vi "LVProjectShortcut_CreateShortcut.vi"(6 "error in":errorcluster, 9 "Wizard":T1) -> (0 "error out":errorcluster, 3 "Cancelled?":bool)   [LabVIEW 2017]
doc: "Use this template to create a wizard dialog."
uses:
  <resource>/Framework/Providers/API/ItemRef.ctl
  <resource>/Framework/Providers/API/mxLvChangeType.ctl
  <resource>/Framework/Providers/API/mxLvUpdateUI.ctl
panel:
  in  "Cancel":bool
  in  "OK Button":bool
  in  "Next":bool
  in  "Name":string caption="Type a name for this shortcut:"
  in  "File Path":path caption="Type the location of the item:"
  out "indication":string
  # "What item would you like to create a shortcut for?"
  # "This wizard helps you to create shortcut to files or folders."
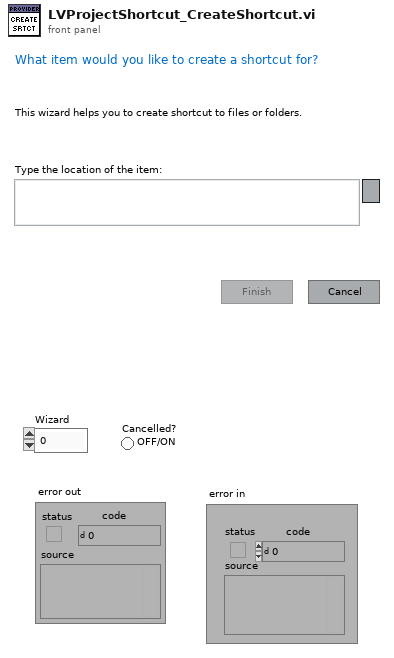
[diagram p1: front panel]
types:
  T1 = typedef "ItemRef.ctl" = u64
  T2 = enum8{"Enabled", "Disabled", "Disabled and Grayed Out"}
  T3 = typedef "mxLvUpdateUI.ctl" = cluster{"Action":u32, "Optional param 1":string, "Optional param 2":i32, "Optional param 3":string}
  T4 = typedef "mxLvChangeType.ctl" = enum32{"Item Created", "Item Modified", "File Modified", "File Deleted", "Item Added", "Item Added to SCC", "Item Renamed", "Item Modified For SCC"}
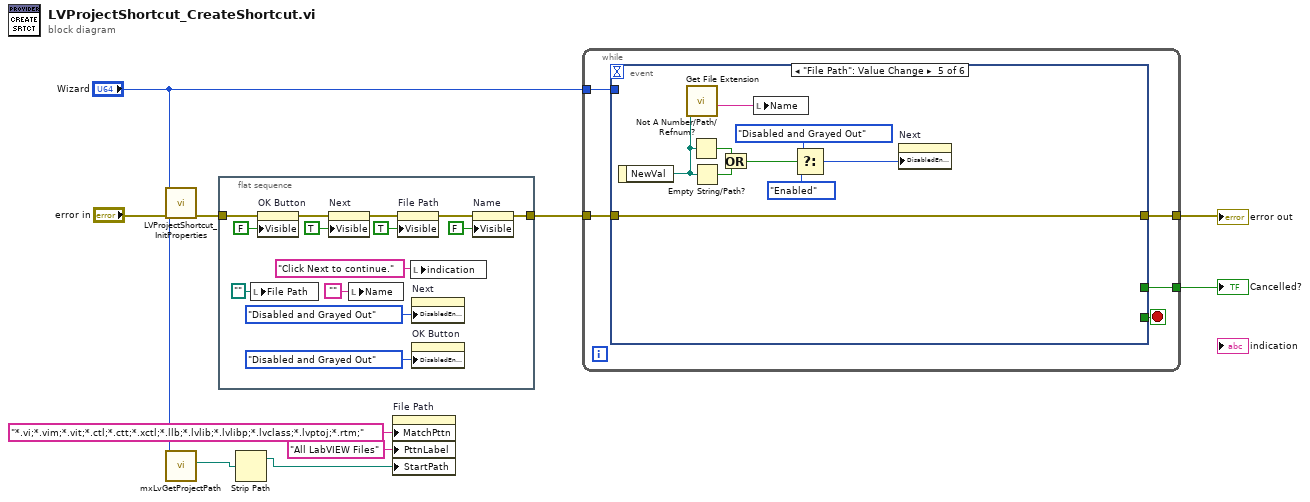
[diagram p0: block diagram]
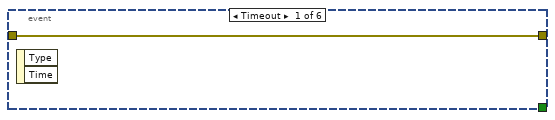
[diagram p2: hidden frame]
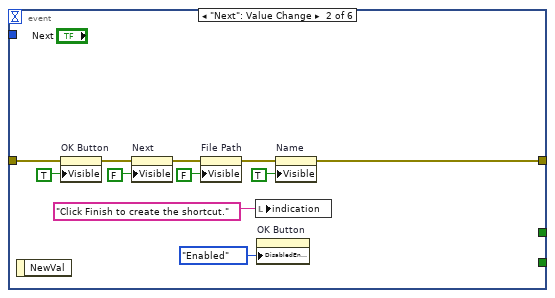
[diagram p3: hidden frame]
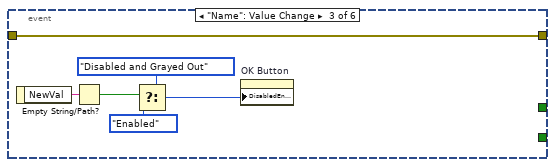
[diagram p4: hidden frame]
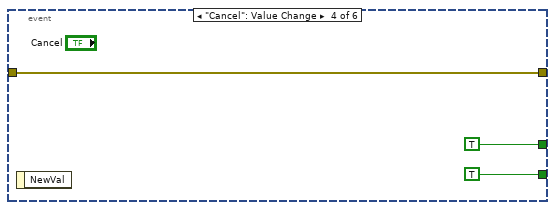
[diagram p5: hidden frame]
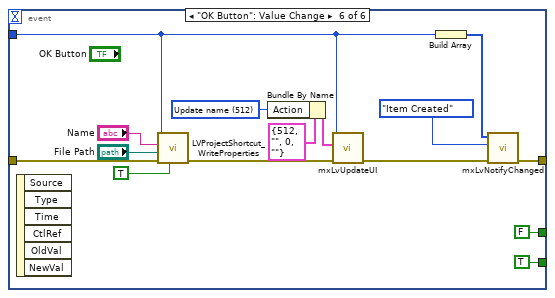
[diagram p6: hidden frame]
diagram:
  n1 = call <resource>:"LVProjectShortcut_InitProperties.vi"("error in"="error in", "Wizard"="Wizard") -> ("error out"=w6:errorcluster)  [unwired: 9 in]
  n2 = call <resource>:"mxLvGetProjectPath.vi"("Item"="Wizard") -> ("Project Path"=w2:path)  [unwired: 8 in, 2 out]
  n3 = flat-sequence {
    tunnel: w6 -> [w16]
    tunnel: [w15] -> w9
    frame #0 {
      n4 = local write "File Path"(path "") -> ()
      n5 = property on="OK Button" class="Bool"(error in=w16, "Visible"=FALSE) -> (error out=w19:errorcluster)  [unwired: 1 in, 1 out]
      n6 = property on="Next" class="Bool"(error in=w19, "Visible"=TRUE) -> (error out=w18:errorcluster)  [unwired: 1 in, 1 out]
      n7 = local write "Name"("") -> ()
      n8 = property on="File Path" class="Path"(error in=w18, "Visible"=TRUE) -> (error out=w17:errorcluster)  [unwired: 1 in, 1 out]
      n9 = local write "indication"("Click Next to continue.") -> ()
      n10 = property on="Next" class="Bool"("DisabledEnum"=T2."Disabled and Grayed Out" ("Disabled")) -> ()  [unwired: 2 in, 2 out]
      n11 = property on="OK Button" class="Bool"("DisabledEnum"=T2."Disabled and Grayed Out" ("Disabled")) -> ()  [unwired: 2 in, 2 out]
      n12 = property on="Name" class="Str"(error in=w17, "Visible"=FALSE) -> (error out=w15:errorcluster)  [unwired: 1 in, 1 out]
    }
  }
  n13 = Strip Path(path=w2) -> (stripped path=w1:path)  [unwired: 1 out]
  n14 = property on="File Path" class="Path"("MatchPttn"="*.vi;*.vim;*.vit;*.ctl;*.ctt;*.xctl;*.llb;*.lvlib;*.lvlibp;*.lvclass;*.lvptoj;*.rtm;" ("Browse Options:Match Pattern"), "PttnLabel"="All LabVIEW Files" ("Browse Options:Pattern Label"), "StartPath"=w1) -> ()  [unwired: 2 in, 2 out]
  n15 = while {
    tunnel: [w28] -> w10
    tunnel: w9 -> [w27]
    tunnel: [w26] -> w8
    tunnel: "Wizard" -> [w25]
    stop <- w29 stop-if-true
    n16 = event shown="[4] \"File Path\": Value Change" {
      selector: _ -> [_ _ _ _ _ _]
      dyn-events: _ -> [_ _ _ _ _ _]
      timeout: _ -> [_ _ _ _ _ _]
      tunnel: [_ _ _ TRUE _ TRUE] -> w29
      tunnel: [_ _ _ TRUE ("Cancelled?") _ FALSE ("Cancelled?")] -> w28
      tunnel: w27 -> [w30 w34 w42 w48 w53 w74]
      tunnel: [w30 w33 w42 w48 w53 w69] -> w26
      tunnel: w25 -> [_ _ _ _ _ w60]
      event Timeout {
        n17 = event-data() -> ()  [unwired: 1 in, 2 out]
      }
      event "Next": Value Change {
        n18 = event-data() -> ()  [unwired: 1 in, 1 out]
        n19 = property on="OK Button" class="Bool"(error in=w34, "Visible"=TRUE) -> (error out=w39:errorcluster)  [unwired: 1 in, 1 out]
        n20 = property on="Next" class="Bool"(error in=w39, "Visible"=FALSE) -> (error out=w40:errorcluster)  [unwired: 1 in, 1 out]
        n21 = property on="File Path" class="Path"(error in=w40, "Visible"=FALSE) -> (error out=w41:errorcluster)  [unwired: 1 in, 1 out]
        n22 = local write "indication"("Click Finish to create the shortcut.") -> ()
        n23 = property on="OK Button" class="Bool"("DisabledEnum"=T2."Enabled" ("Disabled")) -> ()  [unwired: 2 in, 2 out]
        n24 = property on="Name" class="Str"(error in=w41, "Visible"=TRUE) -> (error out=w33:errorcluster)  [unwired: 1 in, 1 out]
      }
      event "Name": Value Change {
        n25 = event-data() -> ("NewVal"=w47:string)  [unwired: 1 in]
        n26 = Empty String/Path?(string/path=w47) -> (empty?=w43:bool)
        n27 = Select(t=T2."Disabled and Grayed Out" ("Disabled"), s=w43, f=T2."Enabled" ("Disabled")) -> (s? t:f=w46:T2)
        n28 = property on="OK Button" class="Bool"("DisabledEnum"=w46) -> ()  [unwired: 2 in, 2 out]
      }
      event "Cancel": Value Change {
        n29 = event-data() -> ()  [unwired: 1 in, 1 out]
      }
      event "File Path": Value Change {
        n30 = event-data() -> ("NewVal"=w52:path)  [unwired: 1 in]
        n31 = call <vilib>:"Get File Extension.vi"("file"=w52) -> ("filename without extension"=w51:string)  [unwired: 6 in, 4 out]
        n32 = Not A Number/Path/Refnum?(number/path/refnum=w52) -> (NaN/Path/Refnum?=w59:bool)
        n33 = Empty String/Path?(string/path=w52) -> (empty?=w58:bool)
        n34 = Or(x=w59, y=w58) -> (x .or. y?=w57:bool)
        n35 = local write "Name"(w51) -> ()
        n36 = Select(t=T2."Disabled and Grayed Out" ("Disabled"), s=w57, f=T2."Enabled" ("Disabled")) -> (s? t:f=w54:T2)
        n37 = property on="Next" class="Bool"("DisabledEnum"=w54) -> ()  [unwired: 2 in, 2 out]
      }
      event "OK Button": Value Change {
        w65 = u32 512 items=["Do nothing"=0, "Browse to item"=1, "Update item state"=2, "Update item icon"=4, "Activate view"=8, "Update view list"=16, "Expand item"=32, "Update child list"=64, "Update help"=128, "Refresh item 'F5'"=256, "Update name"=512, "Update menus and toolbars"=1024, "Update all user interface"=1494] ("Action")
        n38 = event-data() -> ()  [unwired: 1 in, 6 out]
        n39 = call <resource>:"LVProjectShortcut_WriteProperties.vi"("hasPath"=TRUE, "error in"=w74, "filePath"="File Path", "shortcutName"="Name", "Wizard"=w60) -> ("error out"=w64:errorcluster)  [unwired: 6 in]
        n40 = Bundle By Name(cluster=T3 {"Action"=512, "Optional param 1"="", "Optional param 2"=0, "Optional param 3"=""} ("Update UI Settings"), "Action"=w65) -> (w61:T3)
        n41 = call <resource>:"mxLvUpdateUI.vi"("error in"=w64, "Update UI Settings"=w61, "Item"=w60) -> ("error out"=w63:errorcluster)  [unwired: 7 in, 1 out]
        n42 = Build Array(w60) -> (w68:T1[])
        n43 = call <resource>:"mxLvNotifyChanged.vi"("error in (no error)"=w63, "Change Type"=mxLvChangeType."Item Created", "Items"=w68) -> ("error out"=w69:errorcluster)  [unwired: 7 in, 1 out]
      }
    }
  }
  "error out" <- w8
  "Cancelled?" <- w10
